vi "Read Connected_.vi"(8 "error in (no error)":errorcluster, 11 "DatabaseBaseClass in":refnum<class "DatabaseBaseClass.lvclass">) -> (0 "error out":errorcluster, 2 "Connected?":bool, 3 "DatabaseBaseClass out":refnum<class "DatabaseBaseClass.lvclass">)   [LabVIEW 2018, in "Database.lvlib" / "DatabaseBaseClass.lvclass"]
uses:
  DatabaseBaseClass.lvclass
  DatabaseBaseClass.lvclass/DatabaseBaseClass.ctl
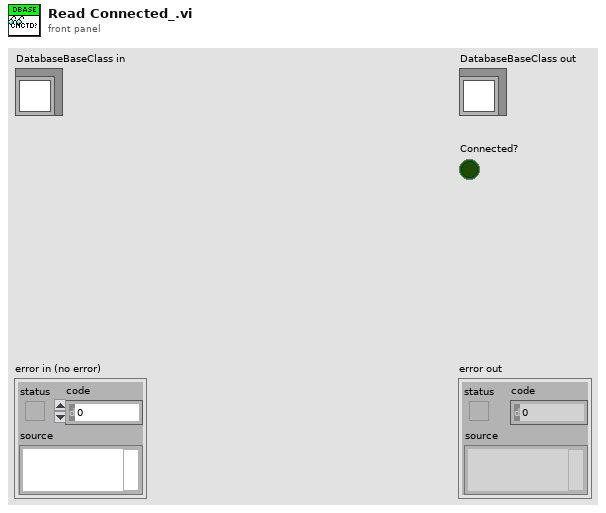
[diagram p1: front panel]
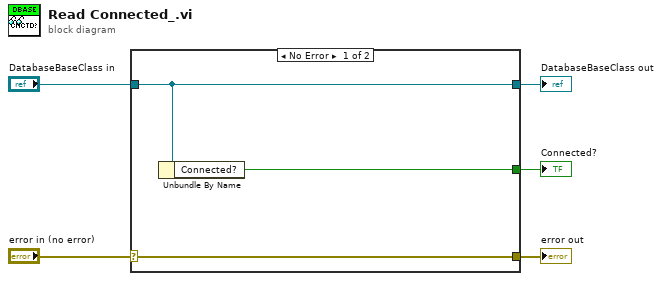
[diagram p0: block diagram]
diagram:
  n1 = case shown="No Error" "error in (no error)" {
    selector: "error in (no error)" -> [w8 w9]
    tunnel: [w8 w9] -> w4
    tunnel: [w7 w10] -> w2
    tunnel: "DatabaseBaseClass in" -> [w7 w10]
    tunnel: [w6 _] -> w1
    frame No Error {
      n2 = Unbundle By Name(w7) -> ("Connected?"=w6:bool)
    }
    frame Error {
    }
  }
  "error out" <- w4
  "DatabaseBaseClass out" <- w2
  "Connected?" <- w1
